vi "HW_GEN - Parse Module Channel Parameters.vi"(8 "error in":errorcluster, 11 "Usedcfg":T3[](array[typedef])) -> (0 "error out":errorcluster, 1 "PhyChUsed[]":bool[](array[boolean]), 2 "InUsedChanIdx[]":i32[](array[numeric]), 3 "AllInUsedModu[]":T2(array[cluster]))   [LabVIEW 2016]
uses:
  Ctrls/HardWare _ Module Configuration.ctl
  Ctrls/HardWare _ Channel Parameters.ctl
  Ctrls/GlobeVaribles.vi
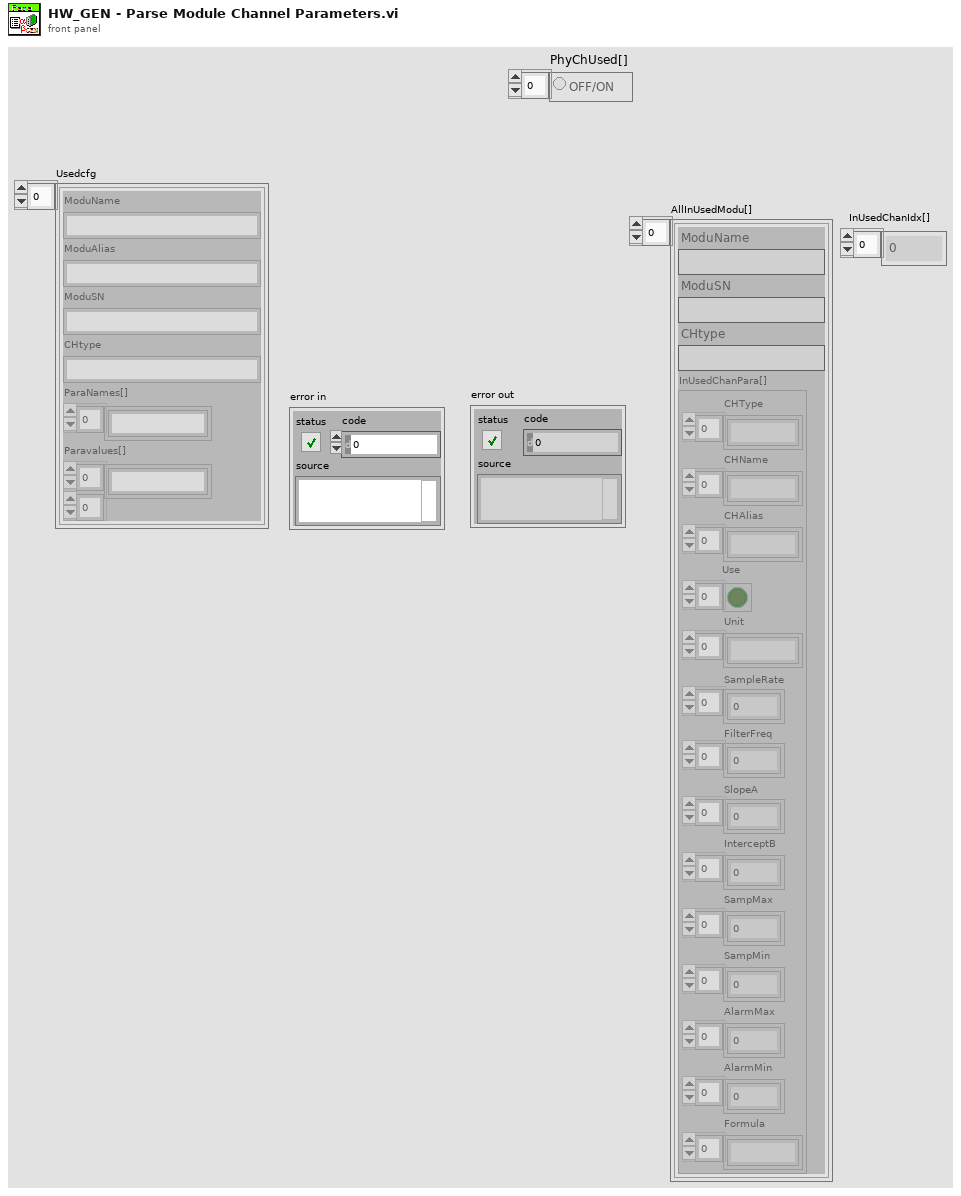
[diagram p1: front panel]
types:
  T1 = typedef "HardWare _ Channel Parameters.ctl" = cluster{"CHType":string[], "CHName":string[], "CHAlias":string[], "Use":bool[], "Unit":string[], "SampleRate":dbl[], "FilterFreq":dbl[], "SlopeA":dbl[], "InterceptB":dbl[], "SampMax":dbl[], "SampMin":dbl[], "AlarmMax":dbl[], "AlarmMin":dbl[], "Formula":string[]}
  T2 = cluster{"ModuName":string, "ModuSN":string, "CHtype":string, "InUsedChanPara[]":T1}[]
  T3 = typedef "HardWare _ Module Configuration.ctl" = cluster{"ModuName":string, "ModuAlias":string, "ModuSN":string, "CHtype":string, "ParaNames[]":string[], "Paravalues[]":string[][]}
  T4 = cluster{"ParaName":string[], "dfltValue":string[]}
  T5 = cluster{string[], string[], string[], bool[], string[], dbl[], dbl[], dbl[], dbl[], dbl[], dbl[], dbl[], dbl[], string[]}
  T6 = cluster{"ModuName":string, "ModuSN":string, "CHtype":string, cluster{string[], string[], string[], bool[], string[], dbl[], dbl[], dbl[], dbl[], dbl[], dbl[], dbl[], dbl[], string[]}}
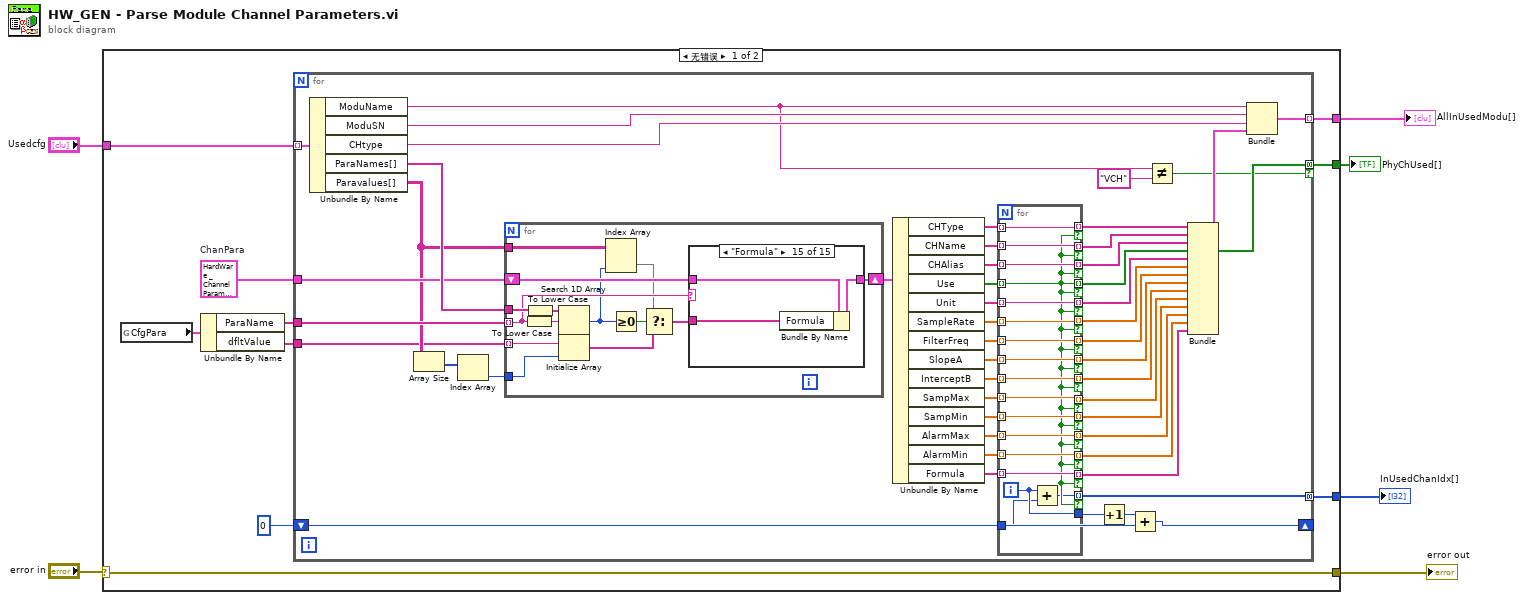
[diagram p0: block diagram]
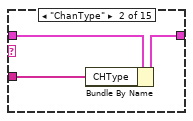
[diagram p3: hidden frame]
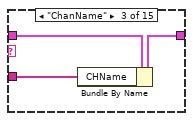
[diagram p4: hidden frame]
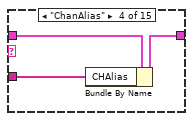
[diagram p5: hidden frame]
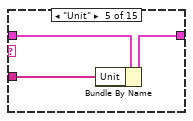
[diagram p6: hidden frame]
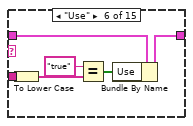
[diagram p7: hidden frame]
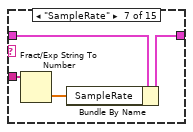
[diagram p8: hidden frame]
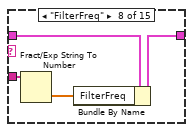
[diagram p9: hidden frame]
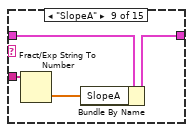
[diagram p10: hidden frame]
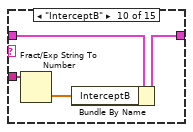
[diagram p11: hidden frame]
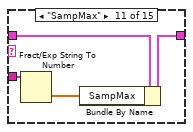
[diagram p12: hidden frame]
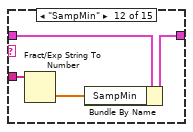
[diagram p13: hidden frame]
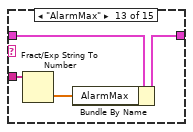
[diagram p14: hidden frame]
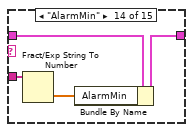
[diagram p15: hidden frame]
diagram:
  n1 = case shown="无错误" "error in" {
    selector: "error in" -> [w14 w151]
    tunnel: "Usedcfg" -> [w16 _]
    tunnel: [w14 w151] -> w4
    tunnel: [w13 _] -> w3
    tunnel: [w8 _] -> w2
    tunnel: [w7 _] -> w1
    frame No Error {
      w15 = T1 {"CHType"=[], "CHName"=[], "CHAlias"=[], "Use"=[], "Unit"=[], "SampleRate"=[], "FilterFreq"=[], "SlopeA"=[], "InterceptB"=[], "SampMax"=[], "SampMin"=[], "AlarmMax"=[], "AlarmMin"=[], "Formula"=[]}  # ChanPara
      n2 = global read "GlobeVaribles.vi" "CfgPara"() -> (w12:T4)
      n3 = Unbundle By Name(w12) -> ("ParaName"=w11:string[], "dfltValue"=w10:string[])
      n4 = for {
        tunnel: w16 -> [w65] mode=indexing
        tunnel: w15 -> [w63]
        tunnel: w11 -> [w62]
        tunnel: w10 -> [w58]
        tunnel: [w30] -> w13 mode=indexing
        shift-right: [w22] -> _
        shift-left: 0 -> [w23]
        tunnel: [w21] -> w8 mode=concatenating
        tunnel: [w20] -> w7 mode=concatenating if=w17
        n5 = Unbundle By Name(w65) -> ("ModuName"=w18:string, "ModuSN"=w29:string, "CHtype"=w28:string, "ParaNames[]"=w64:string[], "Paravalues[]"=w61:string[][])
        n6 = Array Size(array=w61) -> (size(s)=w60:i32[])
        n7 = Index Array(array=w60) -> (element=w59:i32)  [unwired: 1 in]
        n8 = for {
          tunnel: w64 -> [w93]
          shift-right: [w94] -> w57
          shift-left: w63 -> [w96]
          tunnel: w61 -> [w95]
          tunnel: w62 -> [w92] mode=indexing
          tunnel: w59 -> [w89]
          tunnel: w58 -> [w88] mode=indexing
          n9 = To Lower Case(string=w92) -> (all lower case string=w83:string)
          n10 = To Lower Case(string=w93) -> (all lower case string=w84:string[])
          n11 = Search 1D Array(1D array=w84, element=w83) -> (index of element=w85:i32)  [unwired: 1 in]
          n12 = Initialize Array(w88, w89) -> (w87:string[])
          n13 = Index Array(array=w95, index (col)=w85) -> (element=w90:string[])  [unwired: 1 in]
          n14 = Greater Or Equal To 0?(x=w85) -> (x >= 0?=w91:bool)
          n15 = Select(t=w90, s=w91, f=w87) -> (s? t:f=w86:string[])
          n16 = case shown="\"Formula\"" w92 {
            tunnel: w96 -> [w97 w100 w103 w106 w109 w115 w119 w123 w127 w131 w135 w139 w143 w147 w150]
            tunnel: w86 -> [_ w98 w102 w105 w108 w114 w117 w121 w125 w129 w133 w137 w141 w145 w148]
            tunnel: [w97 w99 w101 w104 w107 w113 w118 w122 w126 w130 w134 w138 w142 w146 w149] -> w94
            frame Default {
            }
            frame "ChanType" {
              n17 = Bundle By Name(cluster=w100, "CHType"=w98) -> (w99:T1)
            }
            frame "ChanName" {
              n18 = Bundle By Name(cluster=w103, "CHName"=w102) -> (w101:T1)
            }
            frame "ChanAlias" {
              n19 = Bundle By Name(cluster=w106, "CHAlias"=w105) -> (w104:T1)
            }
            frame "Unit" {
              n20 = Bundle By Name(cluster=w109, "Unit"=w108) -> (w107:T1)
            }
            frame "Use" {
              n21 = To Lower Case(string=w114) -> (all lower case string=w112:string[])
              n22 = Equal?(x="true", y=w112) -> (x = y?=w111:bool[])
              n23 = Bundle By Name(cluster=w115, "Use"=w111) -> (w113:T1)
            }
            frame "SampleRate" {
              n24 = Fract/Exp String To Number(string=w117) -> (number=w116:dbl[])  [unwired: 3 in, 1 out]
              n25 = Bundle By Name(cluster=w119, "SampleRate"=w116) -> (w118:T1)
            }
            frame "FilterFreq" {
              n26 = Fract/Exp String To Number(string=w121) -> (number=w120:dbl[])  [unwired: 3 in, 1 out]
              n27 = Bundle By Name(cluster=w123, "FilterFreq"=w120) -> (w122:T1)
            }
            frame "SlopeA" {
              n28 = Fract/Exp String To Number(string=w125) -> (number=w124:dbl[])  [unwired: 3 in, 1 out]
              n29 = Bundle By Name(cluster=w127, "SlopeA"=w124) -> (w126:T1)
            }
            frame "InterceptB" {
              n30 = Fract/Exp String To Number(string=w129) -> (number=w128:dbl[])  [unwired: 3 in, 1 out]
              n31 = Bundle By Name(cluster=w131, "InterceptB"=w128) -> (w130:T1)
            }
            frame "SampMax" {
              n32 = Fract/Exp String To Number(string=w133) -> (number=w132:dbl[])  [unwired: 3 in, 1 out]
              n33 = Bundle By Name(cluster=w135, "SampMax"=w132) -> (w134:T1)
            }
            frame "SampMin" {
              n34 = Fract/Exp String To Number(string=w137) -> (number=w136:dbl[])  [unwired: 3 in, 1 out]
              n35 = Bundle By Name(cluster=w139, "SampMin"=w136) -> (w138:T1)
            }
            frame "AlarmMax" {
              n36 = Fract/Exp String To Number(string=w141) -> (number=w140:dbl[])  [unwired: 3 in, 1 out]
              n37 = Bundle By Name(cluster=w143, "AlarmMax"=w140) -> (w142:T1)
            }
            frame "AlarmMin" {
              n38 = Fract/Exp String To Number(string=w145) -> (number=w144:dbl[])  [unwired: 3 in, 1 out]
              n39 = Bundle By Name(cluster=w147, "AlarmMin"=w144) -> (w146:T1)
            }
            frame "Formula" {
              n40 = Bundle By Name(cluster=w150, "Formula"=w148) -> (w149:T1)
            }
          }
        }
        n41 = Unbundle By Name(w57) -> ("CHType"=w56:string[], "CHName"=w55:string[], "CHAlias"=w54:string[], "Use"=w33:bool[], "Unit"=w53:string[], "SampleRate"=w52:dbl[], "FilterFreq"=w45:dbl[], "SlopeA"=w51:dbl[], "InterceptB"=w50:dbl[], "SampMax"=w49:dbl[], "SampMin"=w48:dbl[], "AlarmMax"=w47:dbl[], "AlarmMin"=w46:dbl[], "Formula"=w31:string[])
        n42 = for {
          tunnel: w33 -> [w69] mode=indexing
          tunnel: w56 -> [w71] mode=indexing
          tunnel: w55 -> [w72] mode=indexing
          tunnel: w54 -> [w81] mode=indexing
          tunnel: w53 -> [w80] mode=indexing
          tunnel: w52 -> [w79] mode=indexing
          tunnel: w51 -> [w78] mode=indexing
          tunnel: w50 -> [w77] mode=indexing
          tunnel: w49 -> [w76] mode=indexing
          tunnel: w48 -> [w75] mode=indexing
          tunnel: w47 -> [w74] mode=indexing
          tunnel: w46 -> [w82] mode=indexing
          tunnel: [w71] -> w44 mode=indexing if=w69
          tunnel: [w82] -> w35 mode=indexing if=w69
          tunnel: [w72] -> w32 mode=indexing if=w69
          tunnel: [w81] -> w27 mode=indexing if=w69
          tunnel: [w80] -> w43 mode=indexing if=w69
          tunnel: [w79] -> w42 mode=indexing if=w69
          tunnel: [w78] -> w40 mode=indexing if=w69
          tunnel: [w77] -> w39 mode=indexing if=w69
          tunnel: [w76] -> w38 mode=indexing if=w69
          tunnel: [w75] -> w37 mode=indexing if=w69
          tunnel: [w74] -> w36 mode=indexing if=w69
          tunnel: [w69] -> w20 mode=indexing if=w69
          tunnel: w45 -> [w73] mode=indexing
          tunnel: [w73] -> w41 mode=indexing if=w69
          tunnel: w31 -> [w70] mode=indexing
          tunnel: [w70] -> w26 mode=indexing if=w69
          tunnel: [w68] -> w21 mode=indexing if=w69
          tunnel: w23 -> [w66]
          tunnel: [w67] -> w25
          i -> [w67]
          n43 = Add(x=w67, y=w66) -> (x+y=w68:i32)
        }
        n44 = Increment(x=w25) -> (x+1=w24:i32)
        n45 = Add(x=w24, y=w23) -> (x+y=w22:i32)
        n46 = Not Equal?(x=w18, y="VCH" ("x")) -> (x != y?=w17:bool)
        n47 = Bundle(w44, w32, w27, w20, w43, w42, w41, w40, w39, w38, w37, w36, w35, w26) -> (w34:T5)  [unwired: 1 in]
        n48 = Bundle("ModuName"=w18, "ModuSN"=w29, "CHtype"=w28, w34) -> (w30:T6)  [unwired: 1 in]
      }
    }
    frame Error {
    }
  }
  "error out" <- w4
  "AllInUsedModu[]" <- w3
  "InUsedChanIdx[]" <- w2
  "PhyChUsed[]" <- w1
